vi "doKalmanAndMakeFrame.vi"(0 "Vision in":refnum<class "Vision.lvclass">, 1 "Estimador":T7=enum."Nenhum", 2 "cameras array":dbl[](array[numeric]), 5 "Detection Frame":T3 {"robots_blue"."height" format="%+4.3f"; "robots_blue"."pixel_y" format="%+4.3f"; "robots_blue"."pixel_x" format="%+4.3f"; "robots_blue"."orientation" format="%+4.3f"; "robots_blue"."y" format="%+4.3f"; "robots_blue"."confidence" format="%4.3f"; "robots_blue"."x" format="%+4.3f"; "robots_yellow"."height" format="%+4.3f"; "robots_yellow"."pixel_y" format="%+4.3f"; "robots_yellow"."pixel_x" format="%+4.3f"; "robots_yellow"."orientation" format="%+4.3f"; "robots_yellow"."y" format="%+4.3f"; "robots_yellow"."confidence" format="%4.3f"; "robots_yellow"."x" format="%+4.3f"}, 7 "Field":T1, 9 "Fps":dbl=40.0, 10 "Side":enum16{"Esquerdo", "Direito"}(ring)=enum."Direito" caption="Enum", 11 "error in (no error)":errorcluster, 12 "grSim":bool, 13 "max ball vel":dbl, 14 "Team":enum16{"Azul", "Amarelo"}(ring) caption="Enum") -> (4 "Vision out":refnum<class "Vision.lvclass">, 6 "Frame and Field Size out":T2 {"Detection Frame Out"."robots_blue"."height" format="%+4.3f"; "Detection Frame Out"."robots_blue"."pixel_y" format="%+4.3f"; "Detection Frame Out"."robots_blue"."pixel_x" format="%+4.3f"; "Detection Frame Out"."robots_blue"."orientation" format="%+4.3f"; "Detection Frame Out"."robots_blue"."y" format="%+4.3f"; "Detection Frame Out"."robots_blue"."confidence" format="%4.3f"; "Detection Frame Out"."robots_blue"."x" format="%+4.3f"; "Detection Frame Out"."robots_yellow"."height" format="%+4.3f"; "Detection Frame Out"."robots_yellow"."pixel_y" format="%+4.3f"; "Detection Frame Out"."robots_yellow"."pixel_x" format="%+4.3f"; "Detection Frame Out"."robots_yellow"."orientation" format="%+4.3f"; "Detection Frame Out"."robots_yellow"."y" format="%+4.3f"; "Detection Frame Out"."robots_yellow"."confidence" format="%4.3f"; "Detection Frame Out"."robots_yellow"."x" format="%+4.3f"}, 15 "error out":errorcluster)   [LabVIEW 2020, in "Vision.lvclass"]
uses:
  Vision.lvclass
  Old vision/Controls/SSL Detection Frame.ctl
  Old vision/Controls/SSL Detection Robot.ctl
  <vilib>/Analysis/Matrix/Datatypes/RealMatrix.ctl
  Old vision/Controls/SSL Detection Ball.ctl
  Old vision/Controls/Estimadores.ctl
  Old vision/Controls/SSL Field State.ctl
  Robot_class/FieldFIRASim.ctl
  <vilib>/Analysis/Matrix/NI_Matrix.lvlib
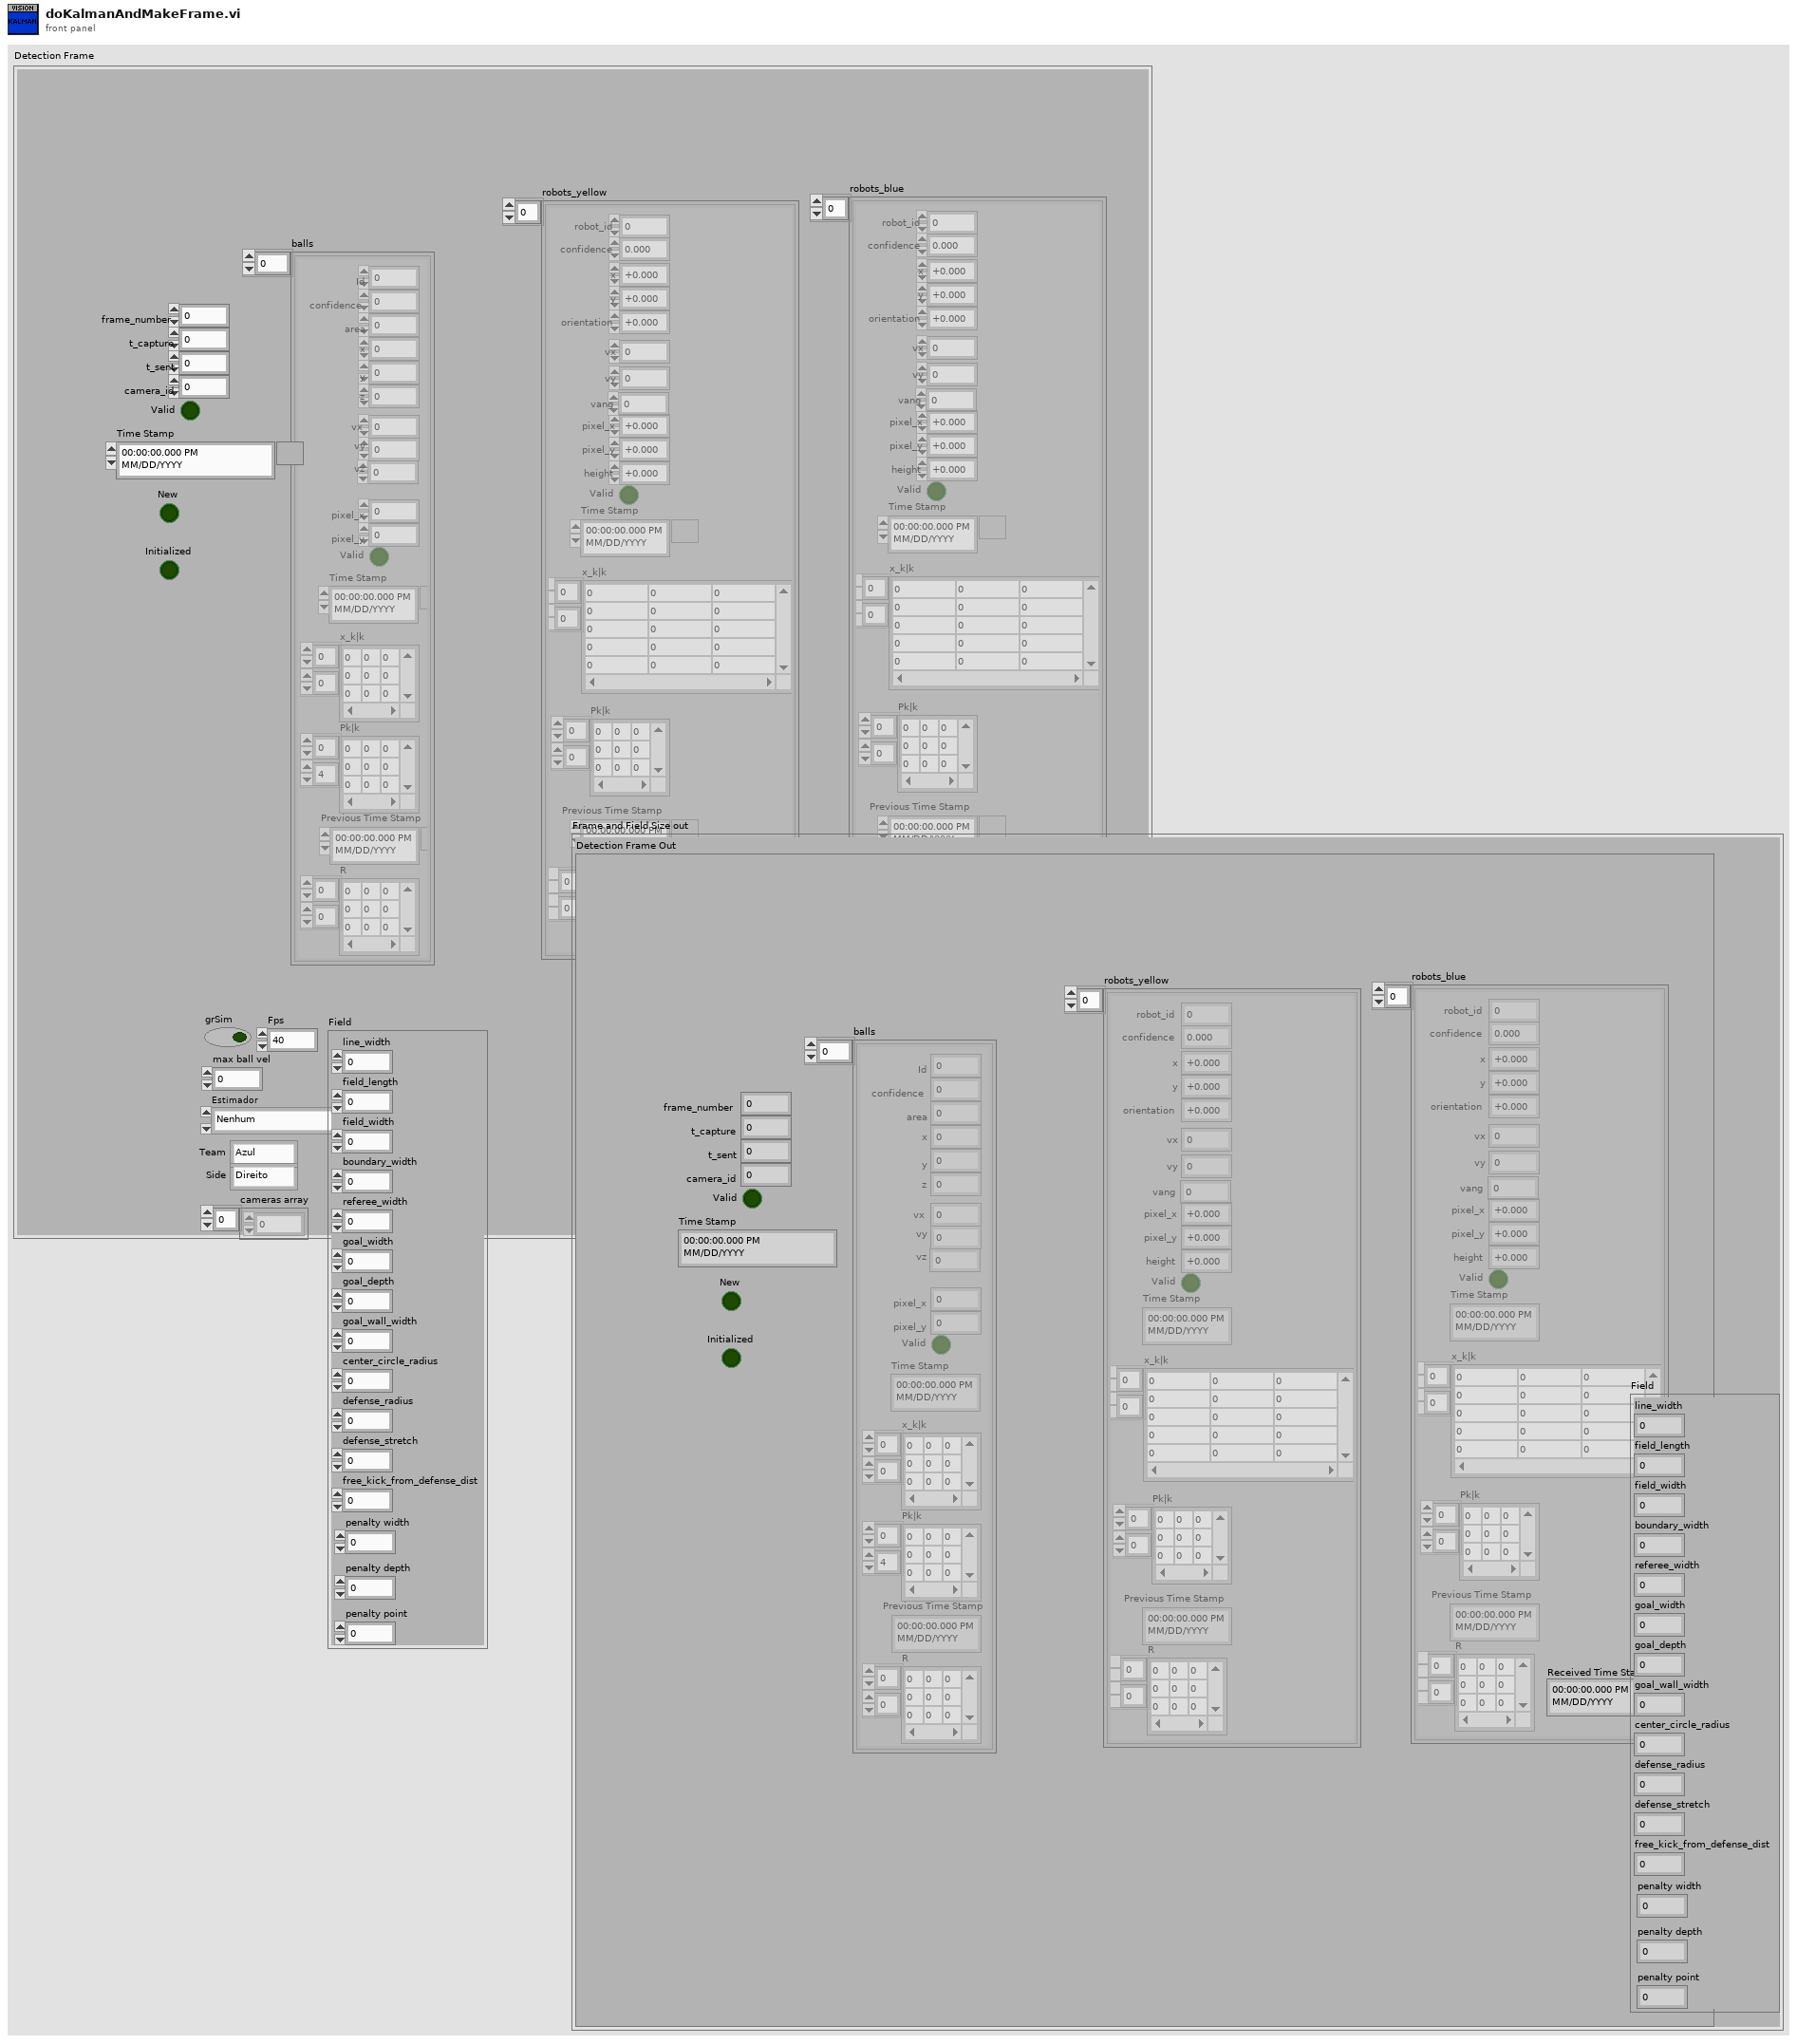
[diagram p1: front panel]
types:
  T1 = typedef "FieldFIRASim.ctl" = cluster{"line_width":u32, "field_length":u32, "field_width":u32, "boundary_width":u32, "referee_width":u32, "goal_width":u32, "goal_depth":u32, "goal_wall_width":u32, "center_circle_radius":u32, "defense_radius":u32, "defense_stretch":u32, "free_kick_from_defense_dist":u32, "penalty width":dbl, "penalty depth":dbl, "penalty point":dbl}
  T2 = typedef "SSL Field State.ctl" = cluster{"Detection Frame Out":T3, "Received Time Stamp":timestamp, "Field ":T1}
  T3 = typedef "SSL Detection Frame.ctl" = cluster{"frame_number":u32, "t_capture":dbl, "t_sent":dbl, "camera_id":u32, "robots_yellow":T4[], "robots_blue":T4[], "balls":T6[], "Valid":bool, "Time Stamp":timestamp, "New":bool, "Initialized":bool}
  T4 = typedef "SSL Detection Robot.ctl" = cluster{"x":sgl, "robot_id":u32, "confidence":sgl, "y":sgl, "orientation":sgl, "pixel_x":sgl, "pixel_y":sgl, "height":sgl, "Valid":bool, "Time Stamp":timestamp, "x_k|k":T5, "Pk|k":T5, "Previous Time Stamp":timestamp, "R":T5, "vx":dbl, "vy":dbl, "vang":dbl}
  T5 = typedef "NI_Matrix.lvlib/RealMatrix.ctl" = dbl[][]
  T6 = typedef "SSL Detection Ball.ctl" = cluster{"x":sgl, "area":u32, "confidence":sgl, "y":sgl, "z":sgl, "pixel_x":sgl, "pixel_y":sgl, "Valid":bool, "Time Stamp":timestamp, "x_k|k":T5, "Pk|k":T5, "Id":u32, "Previous Time Stamp":timestamp, "R":T5, " vx":sgl, "vy":dbl, "vz":dbl}
  T7 = typedef "Estimadores.ctl" = enum16{"4thDerivate", "2ndDerivate", "Nenhum", "Simples", "Kalman"}
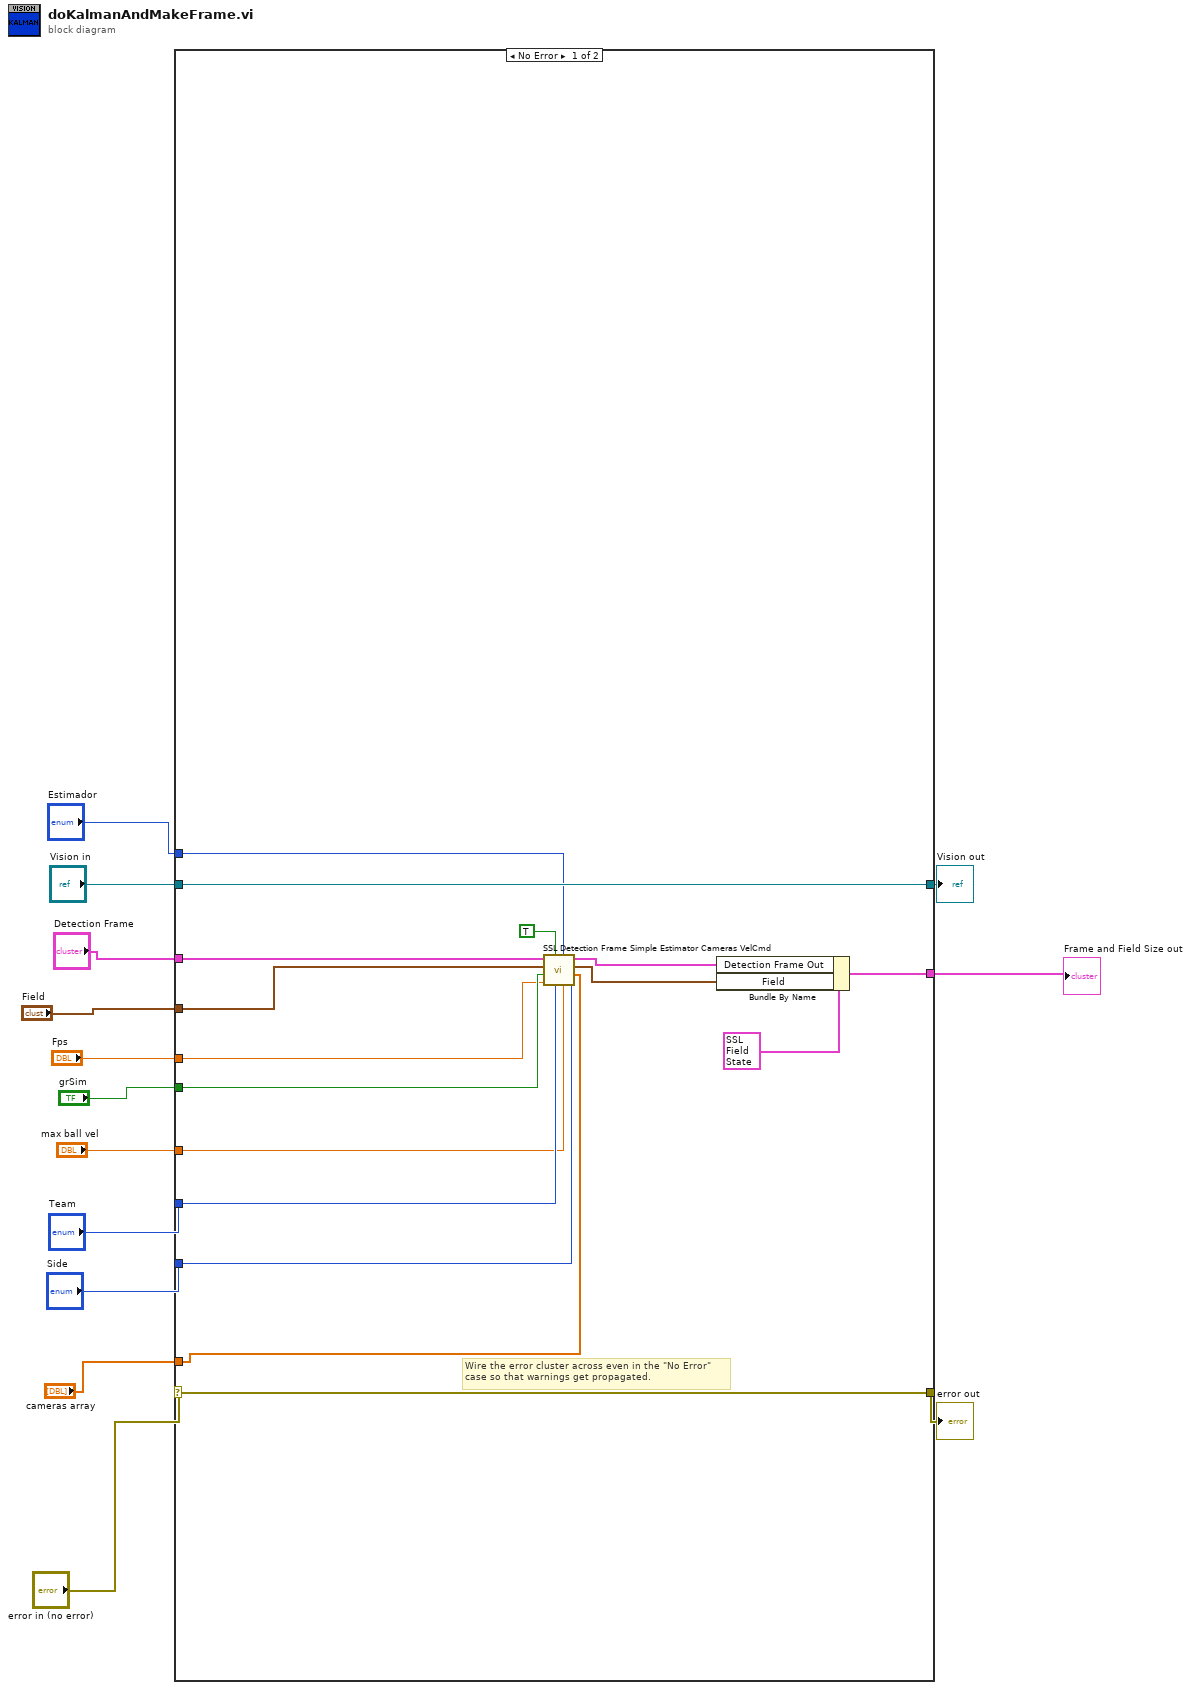
[diagram p0: block diagram]
diagram:
  n1 = case shown="No Error" "error in (no error)" {
    selector: "error in (no error)" -> [w29 w32]
    tunnel: [w29 w32] -> w13
    tunnel: [w30 w31] -> w11
    tunnel: "Vision in" -> [w30 w31]
    tunnel: "Detection Frame" -> [w28 _]
    tunnel: "Field" -> [w27 _]
    tunnel: "Estimador" -> [w26 _]
    tunnel: "Team" -> [w25 _]
    tunnel: "Side" -> [w24 _]
    tunnel: [w21 _] -> w6
    tunnel: "cameras array" -> [w20 _]
    tunnel: "grSim" -> [w19 _]
    tunnel: "Fps" -> [w18 _]
    tunnel: "max ball vel" -> [w17 _]
    frame No Error {
      # "Wire the error cluster across even in the \"No Error\"\ncase so that warnings get propagated."
      n2 = call "SSL Detection Frame Simple Estimator Cameras VelCmd.vi"("Side"=w24, "cameras array"=w20, "max ball vel"=w17, "Estimador"=w26, "Team"=w25, "Enable"=TRUE, "Fps"=w18, "grSim?"=w19, "Field"=w27, "Detection Frame"=w28) -> ("Field"=w15:T1, "Detection Frame Out"=w22:T3)
      n3 = Bundle By Name(cluster=T2 {"Detection Frame Out"={"frame_number"=0, "t_capture"=0.0, "t_sent"=0.0, "camera_id"=0, "robots_yellow"=[], "robots_blue"=[], "balls"=[], "Valid"=FALSE, "Time Stamp"=timestamp(0 s since 1904-01-01), "New"=FALSE, "Initialized"=FALSE}, "Received Time Stamp"=timestamp(0 s since 1904-01-01), "Field "={"line_width"=0, "field_length"=0, "field_width"=0, "boundary_width"=0, "referee_width"=0, "goal_width"=0, "goal_depth"=0, "goal_wall_width"=0, "center_circle_radius"=0, "defense_radius"=0, "defense_stretch"=0, "free_kick_from_defense_dist"=0, "penalty width"=0.0, "penalty depth"=0.0, "penalty point"=0.0}}, "Detection Frame Out"=w22, "Field"=w15) -> (w21:T2)
    }
    frame Error {
    }
  }
  "error out" <- w13
  "Vision out" <- w11
  "Frame and Field Size out" <- w6
